vi "Builds Time Stamp.vi"(1 "Select FORMAT":T1(ring)=enum."00M00D_00h00m", 4 "t0":timestamp) -> (15 "TimeStamp":string)   [LabVIEW 2022 SP3, in "Generic Utilities.lvclass"]
uses:
  Generic Utilities.lvclass
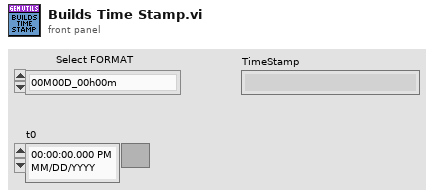
[diagram p1: front panel]
types:
  T1 = enum16{"Y00M00D00h00m00s00", "YYMMDD(hhmmss)", "00Y00M00D00h00m00s", "0000Y00M00D00h00m00s", "00M00D_00h00m", "0000-00-00 00h00m00s", "0000_00_00_00h00m00s", "00000000_000000", "000000_000000", "YYYY-MM-DD,hh:mm:ss"}
  T2 = cluster{"second":i32, "minute":i32, "hour":i32, "day of month":i32, "month":i32, "year":i32, "day of week":i32, "day of year":i32, "is DST":i32}
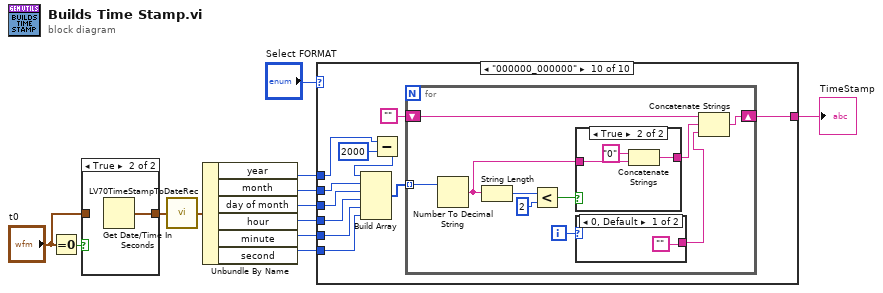
[diagram p0: block diagram]
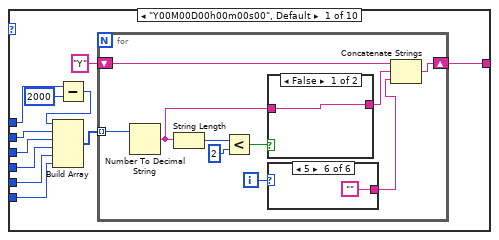
[diagram p3: hidden frame]
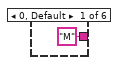
[diagram p4: hidden frame]
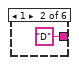
[diagram p5: hidden frame]
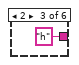
[diagram p6: hidden frame]
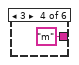
[diagram p7: hidden frame]
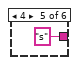
[diagram p8: hidden frame]
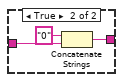
[diagram p9: hidden frame]
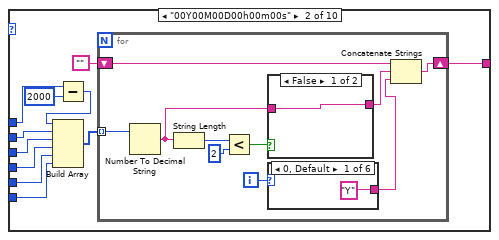
[diagram p10: hidden frame]
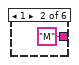
[diagram p11: hidden frame]
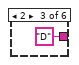
[diagram p12: hidden frame]
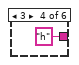
[diagram p13: hidden frame]
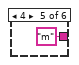
[diagram p14: hidden frame]
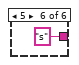
[diagram p15: hidden frame]
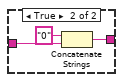
[diagram p16: hidden frame]
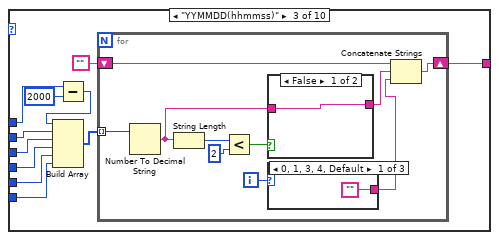
[diagram p17: hidden frame]
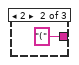
[diagram p18: hidden frame]
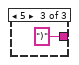
[diagram p19: hidden frame]
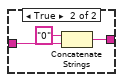
[diagram p20: hidden frame]
diagram:
  n1 = Equal To 0?(x="t0") -> (x = 0?=w2:bool)
  n2 = case shown="True" w2 {
    tunnel: [w13 w14] -> w10
    tunnel: "t0" -> [w13 _]
    frame False {
    }
    frame True {
      n3 = Get Date/Time In Seconds() -> (seconds since 1Jan1904=w14:timestamp)
    }
  }
  n4 = call <vilib>:"LV70TimeStampToDateRec.vi"("time stamp"=w10) -> ("date time rec"=w9:T2)
  n5 = Unbundle By Name(w9) -> ("year"=w8:i32, "month"=w7:i32, "day of month"=w6:i32, "hour"=w5:i32, "minute"=w4:i32, "second"=w3:i32)
  n6 = case shown="\"000000_000000\"" "Select FORMAT" {
    tunnel: w3 -> [w16 w48 w79 w108 _ w162 w191 w220 w249 w276]
    tunnel: w4 -> [w17 w49 w80 w109 w136 w163 w192 w221 w250 w277]
    tunnel: w5 -> [w18 w50 w81 w110 w137 w164 w193 w222 w251 w278]
    tunnel: w6 -> [w23 w54 w85 w111 w138 w165 w194 w223 w252 w279]
    tunnel: w7 -> [w24 w55 w86 w112 w139 w166 w195 w224 w253 w280]
    tunnel: w8 -> [w21 w53 w84 w105 _ w159 w188 w217 w246 w272]
    tunnel: [w15 w47 w78 w107 w135 w161 w190 w219 w248 w275] -> w12
    frame "Y00M00D00h00m00s00", Default {
      n7 = Subtract(x=w21, y=2000) -> (x-y=w19:i32)
      n8 = Build Array(w19, w24, w23, w18, w17, w16) -> (w25:i32[])
      n9 = for {
        tunnel: w25 -> [w31] mode=indexing
        shift-right: [w30] -> w15
        shift-left: "Y" -> [w29]
        i -> [w27]
        n10 = Number To Decimal String(number=w31) -> (decimal integer string=w35:string)  [unwired: 1 out]
        n11 = String Length(string=w35) -> (length=w32:i32)
        n12 = Less?(x=w32, y=2) -> (x < y?=w34:bool)
        n13 = case shown="False" w34 {
          tunnel: w35 -> [w42 w45]
          tunnel: [w42 w43] -> w28
          frame False {
          }
          frame True {
            n14 = Concatenate Strings("0" ("string"), w45) -> (w43:string)
          }
        }
        n15 = case shown="5" w27 {
          tunnel: ["M" "D" "h" "m" "s" ""] -> w26
          frame 0, Default {
          }
          frame 1 {
          }
          frame 2 {
          }
          frame 3 {
          }
          frame 4 {
          }
          frame 5 {
          }
        }
        n16 = Concatenate Strings(w29, w28, w26) -> (w30:string)
      }
    }
    frame "00Y00M00D00h00m00s" {
      n17 = Subtract(x=w53, y=2000) -> (x-y=w51:i32)
      n18 = Build Array(w51, w55, w54, w50, w49, w48) -> (w56:i32[])
      n19 = for {
        tunnel: w56 -> [w62] mode=indexing
        shift-right: [w61] -> w47
        shift-left: "" -> [w60]
        i -> [w58]
        n20 = Number To Decimal String(number=w62) -> (decimal integer string=w66:string)  [unwired: 1 out]
        n21 = String Length(string=w66) -> (length=w63:i32)
        n22 = Less?(x=w63, y=2) -> (x < y?=w65:bool)
        n23 = case shown="False" w65 {
          tunnel: w66 -> [w73 w76]
          tunnel: [w73 w74] -> w59
          frame False {
          }
          frame True {
            n24 = Concatenate Strings("0" ("string"), w76) -> (w74:string)
          }
        }
        n25 = case shown="0, Default" w58 {
          tunnel: ["Y" "M" "D" "h" "m" "s"] -> w57
          frame 0, Default {
          }
          frame 1 {
          }
          frame 2 {
          }
          frame 3 {
          }
          frame 4 {
          }
          frame 5 {
          }
        }
        n26 = Concatenate Strings(w60, w59, w57) -> (w61:string)
      }
    }
    frame "YYMMDD(hhmmss)" {
      n27 = Subtract(x=w84, y=2000) -> (x-y=w82:i32)
      n28 = Build Array(w82, w86, w85, w81, w80, w79) -> (w87:i32[])
      n29 = for {
        tunnel: w87 -> [w93] mode=indexing
        shift-right: [w92] -> w78
        shift-left: "" -> [w91]
        i -> [w89]
        n30 = Number To Decimal String(number=w93) -> (decimal integer string=w97:string)  [unwired: 1 out]
        n31 = String Length(string=w97) -> (length=w94:i32)
        n32 = Less?(x=w94, y=2) -> (x < y?=w96:bool)
        n33 = case shown="False" w96 {
          tunnel: w97 -> [w101 w104]
          tunnel: [w101 w102] -> w90
          frame False {
          }
          frame True {
            n34 = Concatenate Strings("0" ("string"), w104) -> (w102:string)
          }
        }
        n35 = case shown="0, 1, 3, 4, Default" w89 {
          tunnel: ["" "(" ")"] -> w88
          frame 0, 1, 3, 4, Default {
          }
          frame 2 {
          }
          frame 5 {
          }
        }
        n36 = Concatenate Strings(w91, w90, w88) -> (w92:string)
      }
    }
    frame "0000Y00M00D00h00m00s" {
      n37 = Build Array(w105, w112, w111, w110, w109, w108) -> (w113:i32[])
      n38 = for {
        tunnel: w113 -> [w119] mode=indexing
        shift-right: [w118] -> w107
        shift-left: "" -> [w117]
        i -> [w115]
        n39 = Number To Decimal String(number=w119) -> (decimal integer string=w123:string)  [unwired: 1 out]
        n40 = String Length(string=w123) -> (length=w120:i32)
        n41 = Less?(x=w120, y=2) -> (x < y?=w122:bool)
        n42 = case shown="False" w122 {
          tunnel: w123 -> [w130 w133]
          tunnel: [w130 w131] -> w116
          frame False {
          }
          frame True {
            n43 = Concatenate Strings("0" ("string"), w133) -> (w131:string)
          }
        }
        n44 = case shown="0, Default" w115 {
          tunnel: ["Y" "M" "D" "h" "m" "s"] -> w114
          frame 0, Default {
          }
          frame 1 {
          }
          frame 2 {
          }
          frame 3 {
          }
          frame 4 {
          }
          frame 5 {
          }
        }
        n45 = Concatenate Strings(w117, w116, w114) -> (w118:string)
      }
    }
    frame "00M00D_00h00m" {
      n46 = Build Array(w139, w138, w137, w136) -> (w140:i32[])
      n47 = for {
        tunnel: w140 -> [w146] mode=indexing
        shift-right: [w145] -> w135
        shift-left: "" -> [w144]
        i -> [w142]
        n48 = Number To Decimal String(number=w146) -> (decimal integer string=w150:string)  [unwired: 1 out]
        n49 = String Length(string=w150) -> (length=w147:i32)
        n50 = Less?(x=w147, y=2) -> (x < y?=w149:bool)
        n51 = case shown="False" w149 {
          tunnel: w150 -> [w155 w158]
          tunnel: [w155 w156] -> w143
          frame False {
          }
          frame True {
            n52 = Concatenate Strings("0" ("string"), w158) -> (w156:string)
          }
        }
        n53 = case shown="3" w142 {
          tunnel: ["M" "D" "h" "m"] -> w141
          frame 0, Default {
          }
          frame 1 {
          }
          frame 2 {
          }
          frame 3 {
          }
        }
        n54 = Concatenate Strings(w144, w143, w141) -> (w145:string)
      }
    }
    frame "0000-00-00 00h00m00s" {
      n55 = Build Array(w159, w166, w165, w164, w163, w162) -> (w167:i32[])
      n56 = for {
        tunnel: w167 -> [w173] mode=indexing
        shift-right: [w172] -> w161
        shift-left: "" -> [w171]
        i -> [w169]
        n57 = Number To Decimal String(number=w173) -> (decimal integer string=w177:string)  [unwired: 1 out]
        n58 = String Length(string=w177) -> (length=w174:i32)
        n59 = Less?(x=w174, y=2) -> (x < y?=w176:bool)
        n60 = case shown="True" w176 {
          tunnel: w177 -> [w184 w187]
          tunnel: [w184 w185] -> w170
          frame False {
          }
          frame True {
            n61 = Concatenate Strings("0" ("string"), w187) -> (w185:string)
          }
        }
        n62 = case shown="0, Default" w169 {
          tunnel: ["-" "-" " " "h" "m" "s"] -> w168
          frame 0, Default {
          }
          frame 1 {
          }
          frame 2 {
          }
          frame 3 {
          }
          frame 4 {
          }
          frame 5 {
          }
        }
        n63 = Concatenate Strings(w171, w170, w168) -> (w172:string)
      }
    }
    frame "YYYY-MM-DD,hh:mm:ss" {
      n64 = Build Array(w188, w195, w194, w193, w192, w191) -> (w196:i32[])
      n65 = for {
        tunnel: w196 -> [w202] mode=indexing
        shift-right: [w201] -> w190
        shift-left: "" -> [w200]
        i -> [w198]
        n66 = Number To Decimal String(number=w202) -> (decimal integer string=w206:string)  [unwired: 1 out]
        n67 = String Length(string=w206) -> (length=w203:i32)
        n68 = Less?(x=w203, y=2) -> (x < y?=w205:bool)
        n69 = case shown="True" w205 {
          tunnel: w206 -> [w213 w216]
          tunnel: [w213 w214] -> w199
          frame False {
          }
          frame True {
            n70 = Concatenate Strings("0" ("string"), w216) -> (w214:string)
          }
        }
        n71 = case shown="5" w198 {
          tunnel: ["-" "-" "," ":" ":" ""] -> w197
          frame 0, Default {
          }
          frame 1 {
          }
          frame 2 {
          }
          frame 3 {
          }
          frame 4 {
          }
          frame 5 {
          }
        }
        n72 = Concatenate Strings(w200, w199, w197) -> (w201:string)
      }
    }
    frame "0000_00_00_00h00m00s" {
      n73 = Build Array(w217, w224, w223, w222, w221, w220) -> (w225:i32[])
      n74 = for {
        tunnel: w225 -> [w231] mode=indexing
        shift-right: [w230] -> w219
        shift-left: "" -> [w229]
        i -> [w227]
        n75 = Number To Decimal String(number=w231) -> (decimal integer string=w235:string)  [unwired: 1 out]
        n76 = String Length(string=w235) -> (length=w232:i32)
        n77 = Less?(x=w232, y=2) -> (x < y?=w234:bool)
        n78 = case shown="True" w234 {
          tunnel: w235 -> [w242 w245]
          tunnel: [w242 w243] -> w228
          frame False {
          }
          frame True {
            n79 = Concatenate Strings("0" ("string"), w245) -> (w243:string)
          }
        }
        n80 = case shown="2" w227 {
          tunnel: ["_" "_" "_" "h" "m" "s"] -> w226
          frame 0, Default {
          }
          frame 1 {
          }
          frame 2 {
          }
          frame 3 {
          }
          frame 4 {
          }
          frame 5 {
          }
        }
        n81 = Concatenate Strings(w229, w228, w226) -> (w230:string)
      }
    }
    frame "00000000_000000" {
      n82 = Build Array(w246, w253, w252, w251, w250, w249) -> (w254:i32[])
      n83 = for {
        tunnel: w254 -> [w260] mode=indexing
        shift-right: [w259] -> w248
        shift-left: "" -> [w258]
        i -> [w256]
        n84 = Number To Decimal String(number=w260) -> (decimal integer string=w264:string)  [unwired: 1 out]
        n85 = String Length(string=w264) -> (length=w261:i32)
        n86 = Less?(x=w261, y=2) -> (x < y?=w263:bool)
        n87 = case shown="True" w263 {
          tunnel: w264 -> [w267 w270]
          tunnel: [w267 w268] -> w257
          frame False {
          }
          frame True {
            n88 = Concatenate Strings("0" ("string"), w270) -> (w268:string)
          }
        }
        n89 = case shown="0, Default" w256 {
          tunnel: ["" "_"] -> w255
          frame 0, Default {
          }
          frame 2 {
          }
        }
        n90 = Concatenate Strings(w258, w257, w255) -> (w259:string)
      }
    }
    frame "000000_000000" {
      n91 = Subtract(x=w272, y=2000) -> (x-y=w271:i32)
      n92 = Build Array(w271, w280, w279, w278, w277, w276) -> (w281:i32[])
      n93 = for {
        tunnel: w281 -> [w287] mode=indexing
        shift-right: [w286] -> w275
        shift-left: "" -> [w285]
        i -> [w283]
        n94 = Number To Decimal String(number=w287) -> (decimal integer string=w291:string)  [unwired: 1 out]
        n95 = String Length(string=w291) -> (length=w288:i32)
        n96 = Less?(x=w288, y=2) -> (x < y?=w290:bool)
        n97 = case shown="True" w290 {
          tunnel: w291 -> [w294 w297]
          tunnel: [w294 w295] -> w284
          frame False {
          }
          frame True {
            n98 = Concatenate Strings("0" ("string"), w297) -> (w295:string)
          }
        }
        n99 = case shown="0, Default" w283 {
          tunnel: ["" "_"] -> w282
          frame 0, Default {
          }
          frame 2 {
          }
        }
        n100 = Concatenate Strings(w285, w284, w282) -> (w286:string)
      }
    }
  }
  "TimeStamp" <- w12
